vi "ExampleSaveFileToMIDAS.vi"() -> ()   [LabVIEW 2018]
panel:
  out "error out 2":errorcluster
  out "error out":errorcluster
  in  "Filename":string
  in  "File":path
  in  "Request Debug Mode":bool
  in  "MIDAS Sever Port":u16=12345
  in  "MIDAS Server":string="my_midas_server.domain"
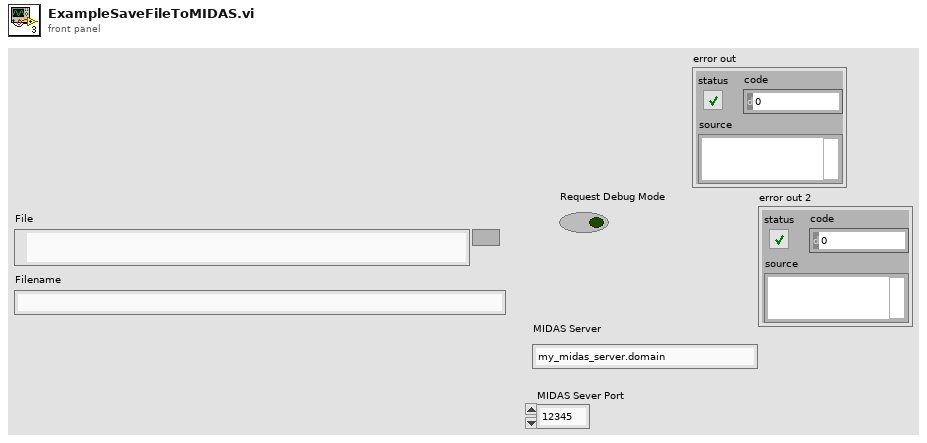
[diagram p1: front panel]
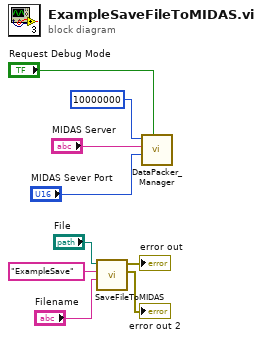
[diagram p0: block diagram]
diagram:
  n1 = call "SaveFileToMIDAS.vi"("Filename"="Filename", "Project Name"="ExampleSave", "File"="File") -> ("error out 2"=→"error out 2":errorcluster, "error out"=→"error out":errorcluster)  [unwired: 7 in]
  n2 = call "DataPacker_Manager.vi"("Request Debug Mode"="Request Debug Mode", "MIDAS Sever Port"="MIDAS Sever Port", "MIDAS Server"="MIDAS Server", "Override Max Event size (Data rate kb/s). Use MIDAS Default = 0"=u32 10000000) -> ()  [unwired: 8 in]
